vi "AWG not-simple.vi"() -> ()   [LabVIEW 2015]
uses:
  <instrlib>/niFgen/niFgen.llb/niFgen Output Mode.ctl
  <instrlib>/niFgen/niFgen.llb/niFgen Create Waveform (WDT).vi
panel:
  in  "Element":enum32{"Radio Selection 1", "Radio Selection 2"}(radio)
  in  "Save Current Waveform":bool
  in  "Load Saved Waveform":bool
  in  "Stable  Measurement":bool
  in  "Stable 2":sgl(slide) min=0 max=10 step=0.001 scale=0.0..10.0
  in  "Stable":sgl(slide) min=0 max=10 step=0.001 scale=0.0..10.0
  in  "Rare":sgl(slide) min=0 max=10 step=0.001 scale=0.0..10.0
  in  "Tab Control":T1(tab)
  in  "Calculate Rare \nFrom Stable":bool
  in  "Stop 2":bool
  in  "Apply Settings":bool
  out "Waveform Chart 3":waveform(dbl)(graph)
  in  "Tuning Isotope":enum32{"Stable 1", "Stable 2", "Rare"}(radio)
  in  "Stable 2 window (ms)":dbl=0.1
  out "Stable 2 Samples":dbl
  in  "Create New Waveform":bool
  out "Waveform Chart 2":waveform(dbl)(graph)
  in  "Bounce Field Frequency (Hz)":dbl=10.0
  in  "Waveform Samples":dbl=100000.0
  out "Waveform Period (ms)":dbl
  out "Waveform File Size (MB)":dbl
  in  "Stable window (ms)":dbl=0.1
  out "Rare Window (ms)":dbl
  out "Stable Samples":dbl
  out "Rare Samples":dbl
  out "delta-T":dbl
  in  "Stop":bool
  in  "Apply Changes":bool
  out "Sample Rate":dbl
  in  "Resource Name":refnum<k15>="ArbWaveformGen"
  out "Error Report":errorcluster
  in  "User Gain":dbl=10.0
  in  "FGEN Gain":dbl=5.0
  in  "Bytes/Sample":dbl=2.0
  # "Stable - Stable"
  # "Single Stable"
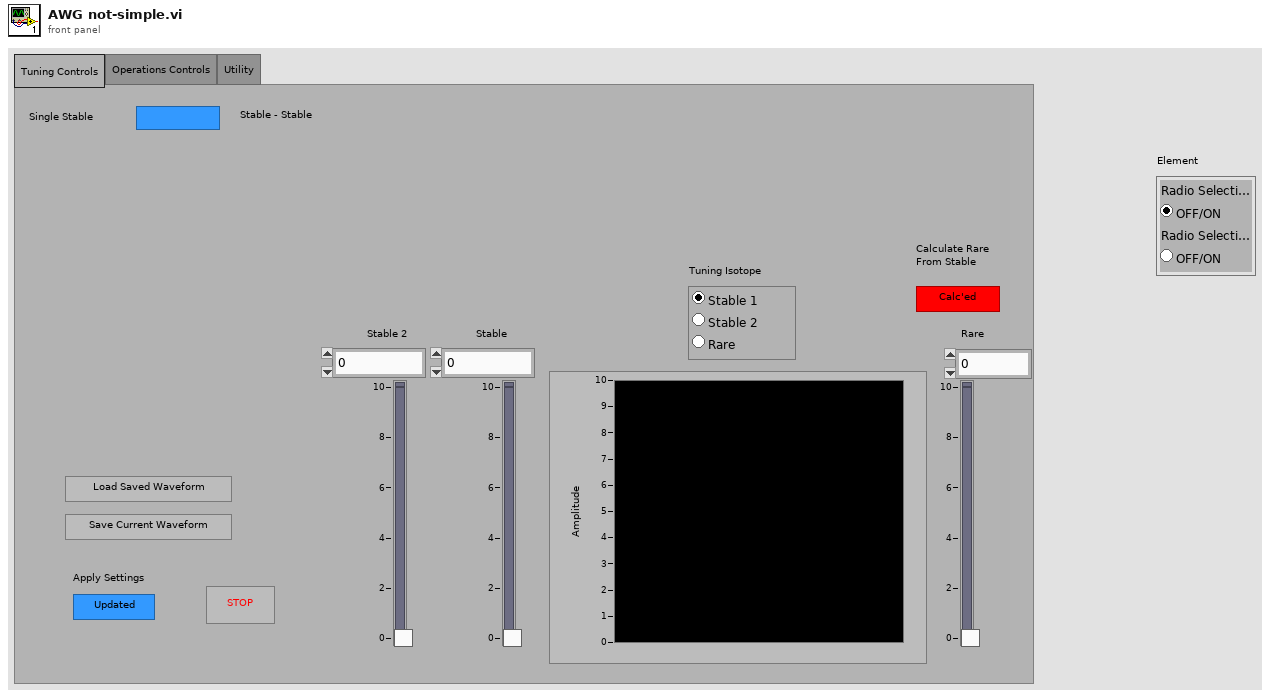
[diagram p1: front panel]
types:
  T1 = enum32{"Tuning Controls", "Operations Controls", "Utility"}
  T2 = enum8{"Enabled", "Disabled", "Disabled and Grayed Out"}
  T3 = typedef "niFgen Output Mode.ctl" = u32
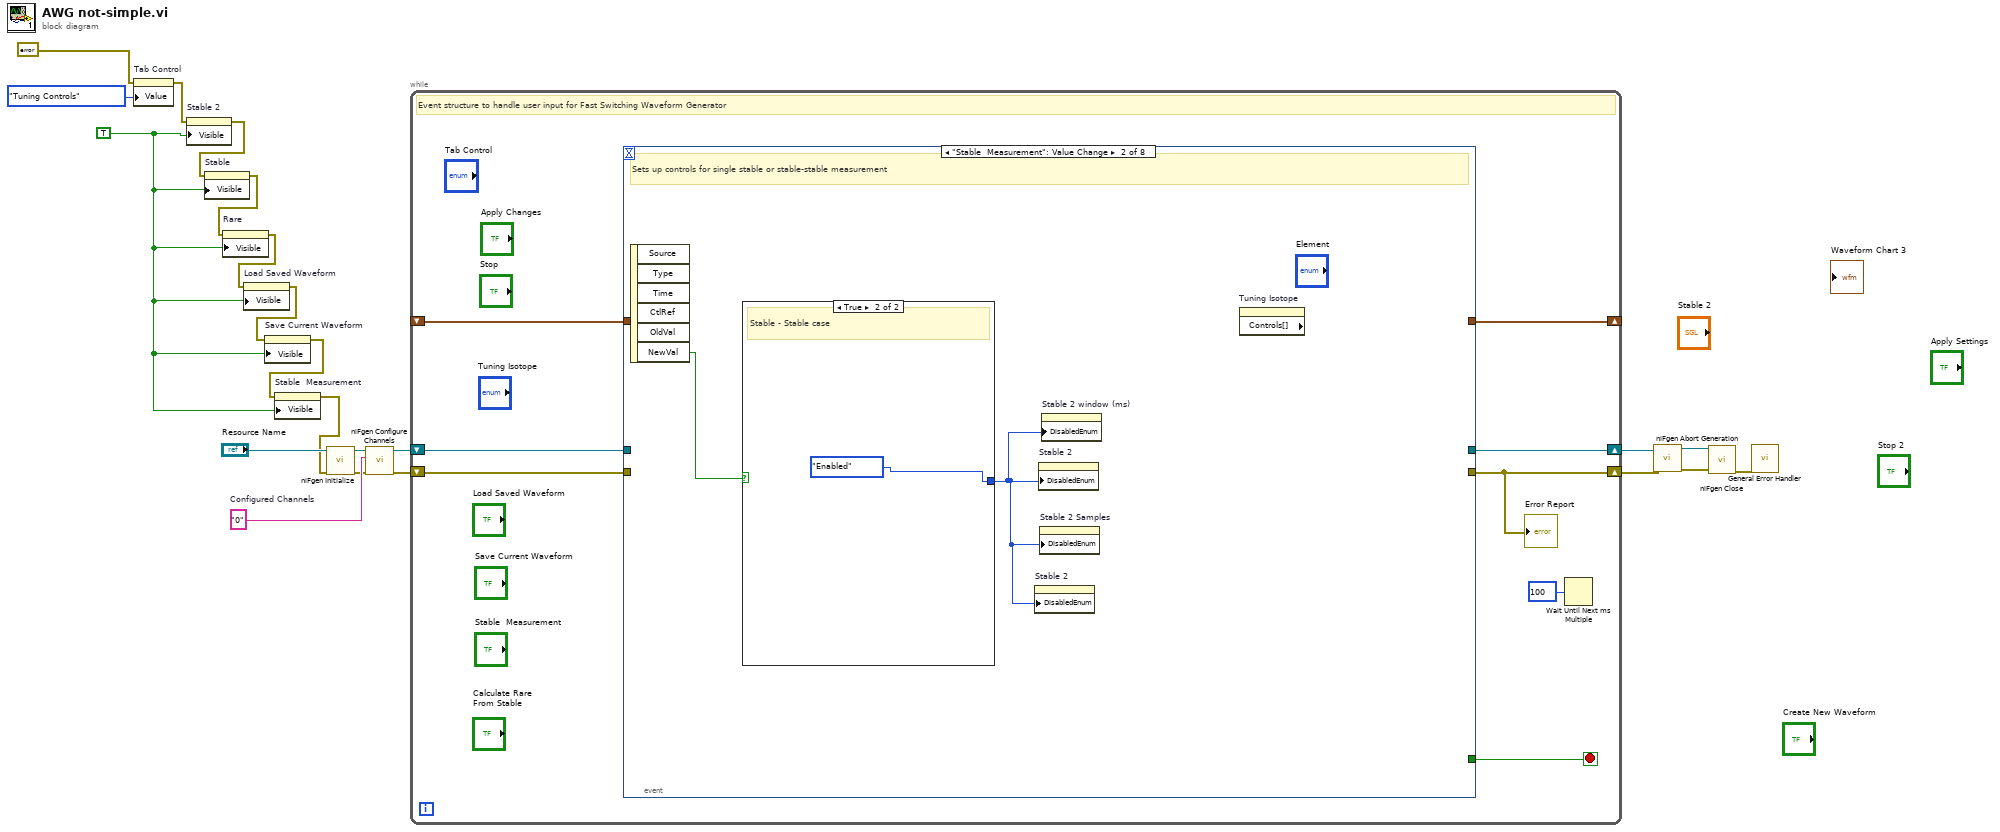
[diagram p0: block diagram]
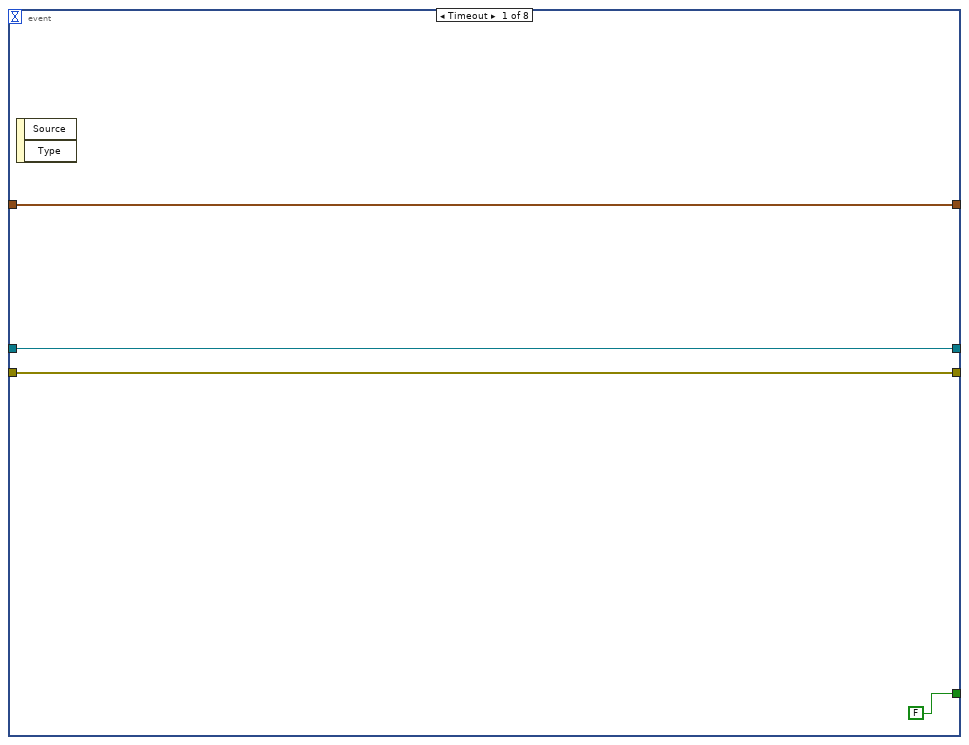
[diagram p2: hidden frame]
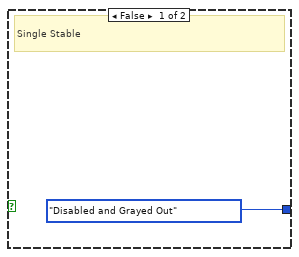
[diagram p3: hidden frame]
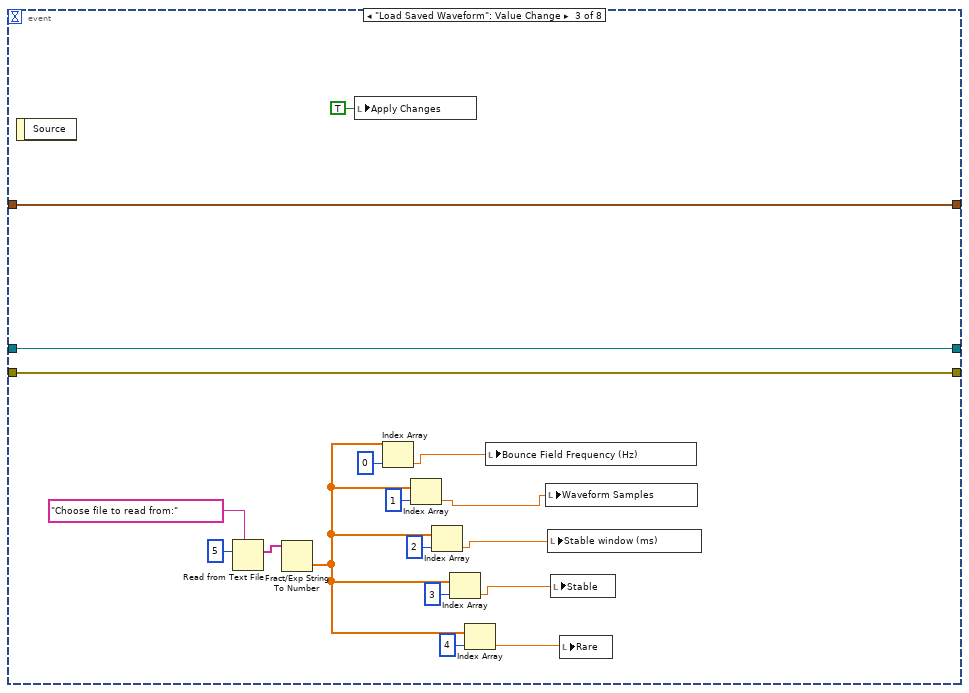
[diagram p4: hidden frame]
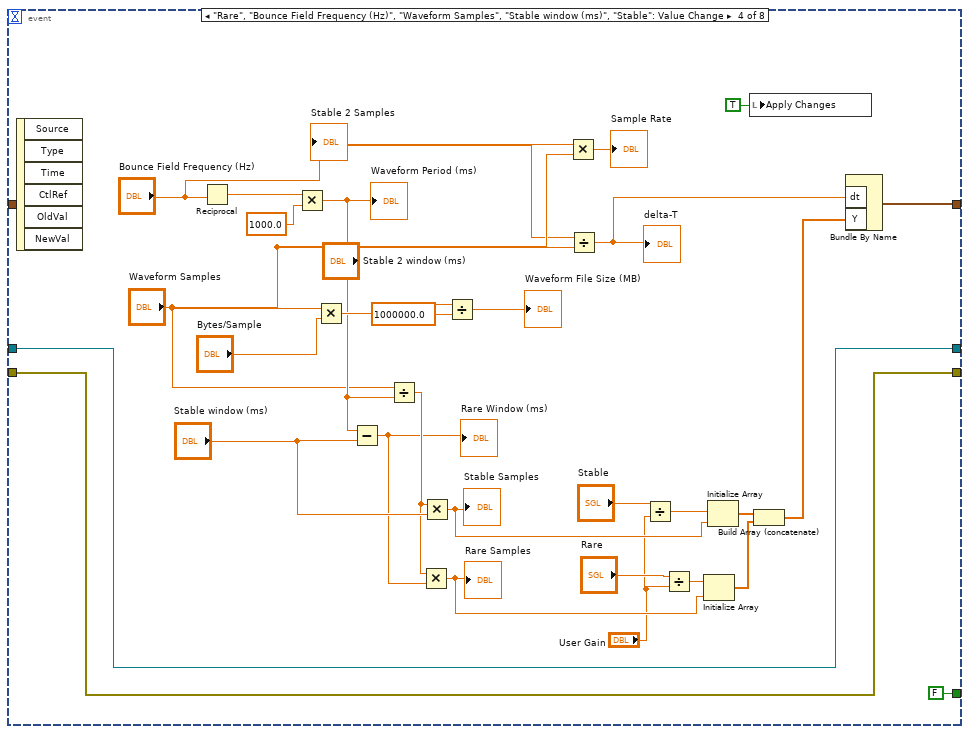
[diagram p5: hidden frame]
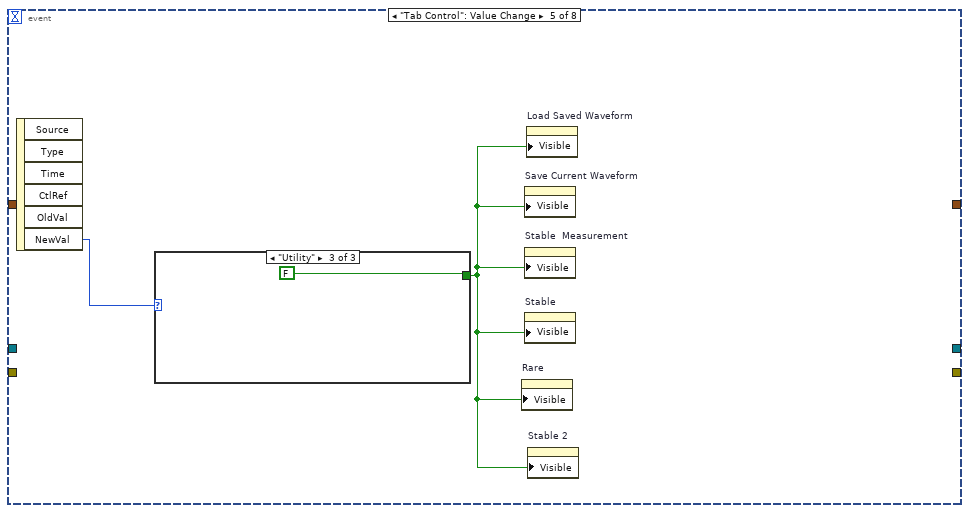
[diagram p6: hidden frame]
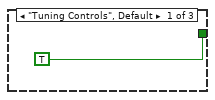
[diagram p7: hidden frame]
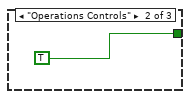
[diagram p8: hidden frame]
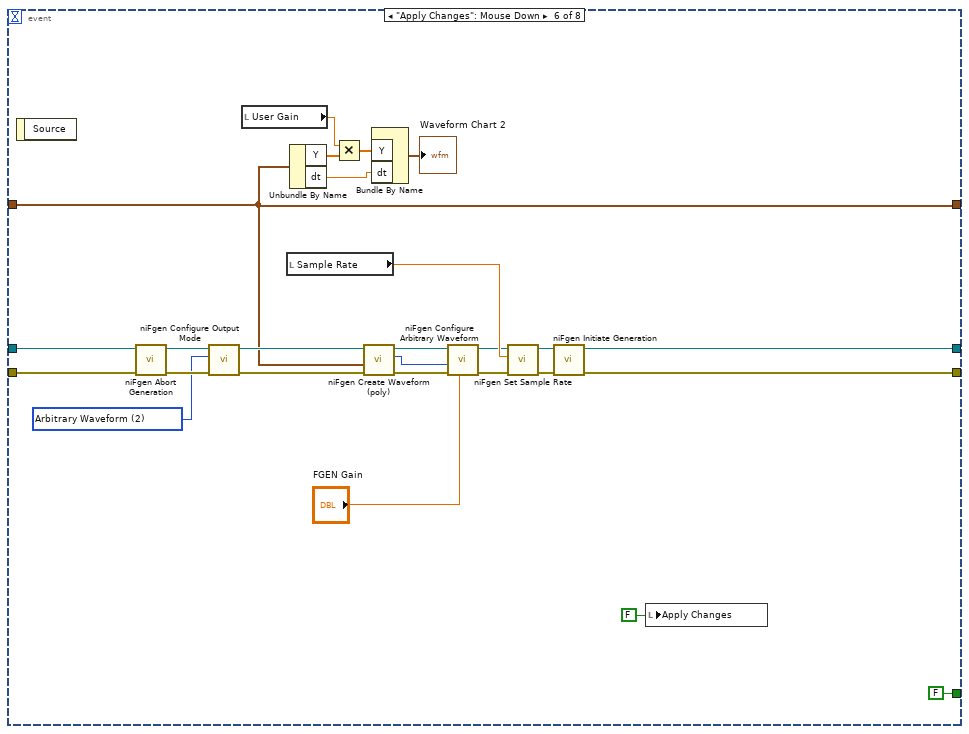
[diagram p9: hidden frame]
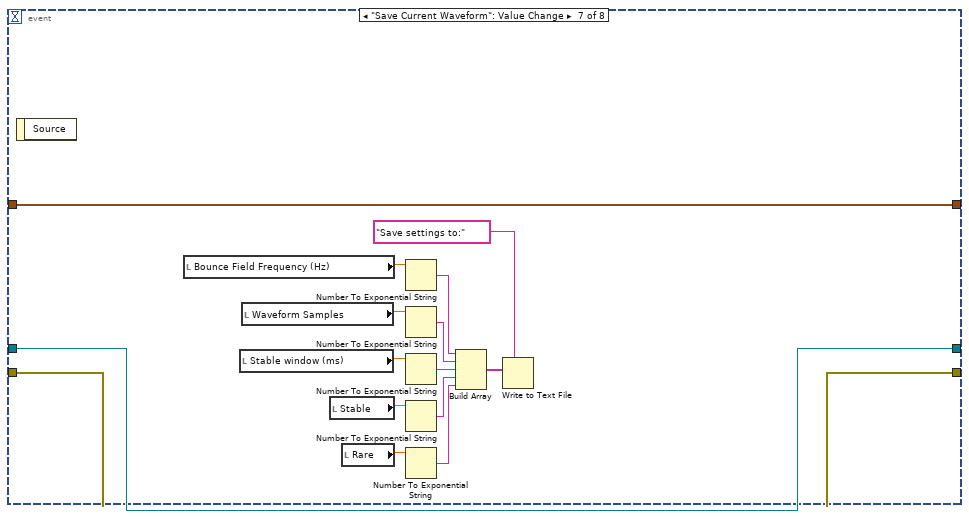
[diagram p10: hidden frame]
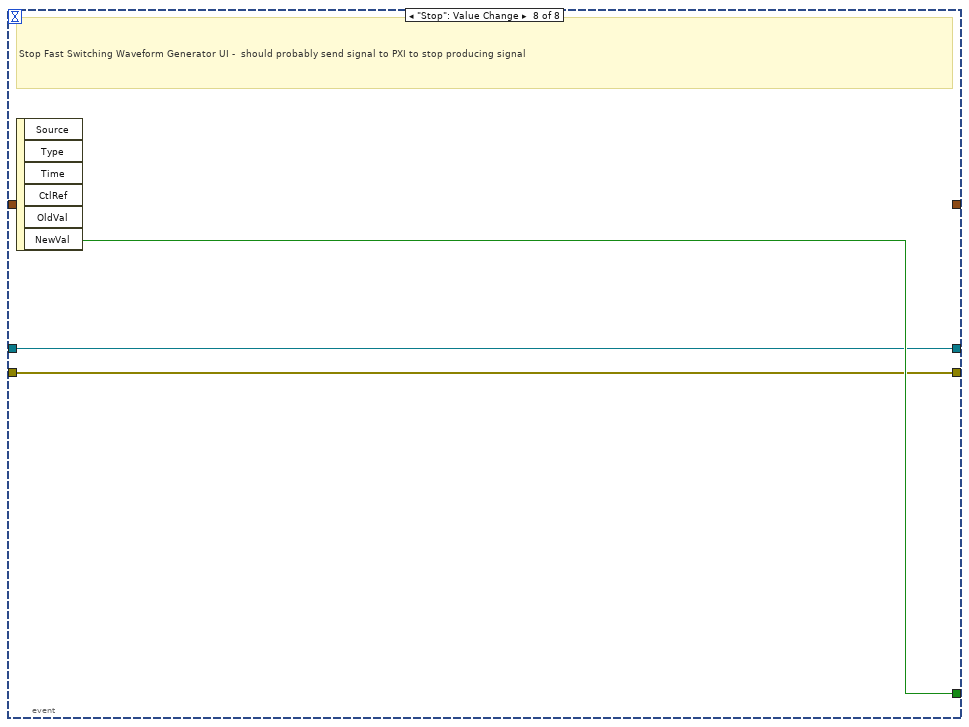
[diagram p11: hidden frame]
diagram:
  w1 = TRUE
  w20 = "0"  # Configured Channels
  n1 = property on="Tab Control" class="TabCtl (strict)"(error in=errorcluster {"status"=FALSE, "code"=0, "source"=""} ("error in (no error)"), "Value"=T1."Tuning Controls" ("Tab Control")) -> (error out=w7:errorcluster)  [unwired: 1 in, 1 out]
  n2 = property on="Stable 2" class="Slide (strict)"(error in=w7, "Visible"=w1) -> (error out=w6:errorcluster)  [unwired: 1 in, 1 out]
  n3 = property on="Stable" class="Slide (strict)"(error in=w6, "Visible"=w1) -> (error out=w5:errorcluster)  [unwired: 1 in, 1 out]
  n4 = property on="Rare" class="Slide (strict)"(error in=w5, "Visible"=w1) -> (error out=w4:errorcluster)  [unwired: 1 in, 1 out]
  n5 = property on="Load Saved Waveform" class="Bool"(error in=w4, "Visible"=w1) -> (error out=w3:errorcluster)  [unwired: 1 in, 1 out]
  n6 = property on="Save Current Waveform" class="Bool"(error in=w3, "Visible"=w1) -> (error out=w2:errorcluster)  [unwired: 1 in, 1 out]
  n7 = property on="Stable  Measurement" class="Bool (strict)"(error in=w2, "Visible"=w1) -> (error out=w10:errorcluster)  [unwired: 1 in, 1 out]
  n8 = call <instrlib>:"niFgen Initialize.vi"("error in (no error)"=w10, "Resource Name"="Resource Name") -> ("error out"=w19:errorcluster, "Instrument Handle Out"=w18:refnum<k15>)  [unwired: 8 in]
  n9 = call <instrlib>:"niFgen Configure Channels.vi"("error in (no error)"=w19, "Channels"=w20, "Instrument Handle"=w18) -> ("error out"=w15:errorcluster, "Instrument Handle Out"=w16:refnum<k15>)  [unwired: 7 in]
  n10 = while {
    shift-right: [w29] -> _
    shift-left: _ -> [w28]
    shift-right: [w22] -> w14
    shift-left: w16 -> [w24]
    shift-right: [w23] -> w13
    shift-left: w15 -> [w25]
    stop <- w26 stop-if-true
    # "Event structure to handle user input for Fast Switching Waveform Generator"
    n11 = event shown="[1] \"Stable  Measurement\": Value Change" {
      selector: _ -> [_ _ _ _ _ _ _ _]
      dyn-events: _ -> [_ _ _ _ _ _ _ _]
      timeout: _ -> [_ _ _ _ _ _ _ _]
      tunnel: [w33 _ w40 w69 _ w95 w130 _] -> w29
      tunnel: w28 -> [w33 _ w40 _ _ w95 w130 _]
      tunnel: [FALSE ("NewVal") _ _ FALSE ("stop") _ FALSE ("stop") _ w133] -> w26
      tunnel: w25 -> [w30 _ w38 w66 _ w99 w117 w132]
      tunnel: w24 -> [w31 _ w39 w65 _ w100 w116 w131]
      tunnel: [w30 _ w38 w66 _ w113 w117 w132] -> w23
      tunnel: [w31 _ w39 w65 _ w112 w116 w131] -> w22
      event Timeout {
        n12 = event-data() -> ()  [unwired: 1 in, 2 out]
      }
      event "Stable  Measurement": Value Change {
        # "Sets up controls for single stable or stable-stable measurement"
        n13 = event-data() -> ("NewVal"=w35:bool)  [unwired: 1 in, 5 out]
        n14 = case shown="True" w35 {
          tunnel: [T2."Disabled and Grayed Out" ("Disabled") T2."Enabled" ("Disabled")] -> w34
          frame False {
            # "Single Stable"
          }
          frame True {
            # "Stable - Stable case"
          }
        }
        n15 = property on="Stable 2" class="Bool (strict)"("DisabledEnum"=w34) -> ()  [unwired: 2 in, 2 out]
        n16 = property on="Stable 2" class="Slide (strict)"("DisabledEnum"=w34) -> ()  [unwired: 2 in, 2 out]
        n17 = property on="Stable 2 Samples" class="DigNum (strict)"("DisabledEnum"=w34) -> ()  [unwired: 2 in, 2 out]
        n18 = property on="Stable 2 window (ms)" class="DigNum (strict)"("DisabledEnum"=w34) -> ()  [unwired: 2 in, 2 out]
        n19 = property on="Tuning Isotope" class="RadioBtnsControl (strict)" props=["Controls[]"]() -> ()  [unwired: 2 in, 3 out]
      }
      event "Load Saved Waveform": Value Change {
        n20 = event-data() -> ()  [unwired: 1 in, 1 out]
        n21 = Read from Text File(prompt (Open existing file)="Choose file to read from:", count=5) -> (text=w53:string[])  [unwired: 2 in, 3 out]
        n22 = Fract/Exp String To Number(string=w53) -> (number=w46:dbl[])  [unwired: 3 in, 1 out]
        n23 = local write "Apply Changes"(TRUE ("Apply Changes")) -> ()
        n24 = Index Array(array=w46, index=0) -> (element=w51:dbl)
        n25 = Index Array(array=w46, index=1) -> (element=w47:dbl)
        n26 = Index Array(array=w46, index=2) -> (element=w48:dbl)
        n27 = Index Array(array=w46, index=3) -> (element=w49:dbl)
        n28 = Index Array(array=w46, index=4) -> (element=w50:dbl)
        n29 = local write "Bounce Field Frequency (Hz)"(w51) -> ()
        n30 = local write "Waveform Samples"(w47) -> ()
        n31 = local write "Stable window (ms)"(w48) -> ()
        n32 = local write "Stable"(w49) -> ()
        n33 = local write "Rare"(w50) -> ()
      }
      event "Rare", "Bounce Field Frequency (Hz)", "Waveform Samples", "Stable window (ms)", "Stable": Value Change {
        n34 = event-data() -> ()  [unwired: 1 in, 6 out]
        n35 = Reciprocal(x="Bounce Field Frequency (Hz)") -> (1/x=w64:dbl)
        n36 = Multiply(x=w64, y=1000.0) -> (x*y=w72:dbl)
        "Waveform Period (ms)" <- w72
        n37 = Multiply(x="Waveform Samples", y="Bytes/Sample") -> (x*y=w79:dbl)
        n38 = Subtract(x=w72, y="Stable window (ms)") -> (x-y=w81:dbl)
        "Rare Window (ms)" <- w81
        n39 = Divide(x="Waveform Samples", y=w72) -> (x/y=w82:dbl)
        n40 = Multiply(x=w82, y=w81) -> (x*y=w75:dbl)
        "Rare Samples" <- w75
        n41 = Multiply(x=w82, y="Stable window (ms)") -> (x*y=w76:dbl)
        "Stable Samples" <- w76
        n42 = Divide(x=w79, y=1000000.0) -> (x/y=→"Waveform File Size (MB)":dbl)
        n43 = Multiply(x="Bounce Field Frequency (Hz)", y="Waveform Samples") -> (x*y=→"Sample Rate":dbl)
        n44 = Divide(x="Bounce Field Frequency (Hz)", y="Waveform Samples") -> (x/y=w70:dbl)
        "delta-T" <- w70
        n45 = Divide(x="Stable", y="User Gain") -> (x/y=w61:dbl)
        n46 = Divide(x="Rare", y="User Gain") -> (x/y=w59:dbl)
        n47 = Initialize Array(w59, w75) -> (w73:dbl[])
        n48 = Initialize Array(w61, w76) -> (w74:dbl[])
        n49 = local write "Apply Changes"(TRUE ("Apply Changes")) -> ()
        n50 = Build Array (concatenate)(w74, w73) -> (w71:dbl[])
        n51 = Bundle By Name("dt"=w70, "Y"=w71) -> (w69:waveform(dbl))  [unwired: 1 in]
      }
      event "Tab Control": Value Change {
        n52 = event-data() -> ("NewVal"=w86:T1)  [unwired: 1 in, 5 out]
        n53 = case shown="\"Utility\"" w86 {
          tunnel: [TRUE ("Visible") TRUE ("Visible") FALSE ("Visible")] -> w85
          frame "Tuning Controls", Default {
          }
          frame "Operations Controls" {
          }
          frame "Utility" {
          }
        }
        n54 = property on="Rare" class="Slide (strict)"("Visible"=w85) -> ()  [unwired: 2 in, 2 out]
        n55 = property on="Save Current Waveform" class="Bool"("Visible"=w85) -> ()  [unwired: 2 in, 2 out]
        n56 = property on="Stable  Measurement" class="Bool (strict)"("Visible"=w85) -> ()  [unwired: 2 in, 2 out]
        n57 = property on="Stable" class="Slide (strict)"("Visible"=w85) -> ()  [unwired: 2 in, 2 out]
        n58 = property on="Load Saved Waveform" class="Bool"("Visible"=w85) -> ()  [unwired: 2 in, 2 out]
        n59 = property on="Stable 2" class="Slide (strict)"("Visible"=w85) -> ()  [unwired: 2 in, 2 out]
      }
      event "Apply Changes": Mouse Down {
        w101 = T3 2 items=["Standard Function", "Frequency List", "Arbitrary Waveform", "Arbitrary Sequence", "Script"] ("Output Mode (default: 0=Standard Function)")
        n60 = event-data() -> ()  [unwired: 1 in, 1 out]
        n61 = call <instrlib>:"niFgen Abort Generation.vi"("error in (no error)"=w99, "Instrument Handle"=w100) -> ("error out"=w102:errorcluster, "Instrument Handle Out"=w103:refnum<k15>)  [unwired: 8 in]
        n62 = call <instrlib>:"niFgen Configure Output Mode.vi"("error in (no error)"=w102, "Output Mode (default: 0=Standard Function)"=w101, "Instrument Handle"=w103) -> ("error out"=w97:errorcluster, "Instrument Handle Out"=w98:refnum<k15>)  [unwired: 6 in]
        n63 = local read "User Gain"() -> (w91:dbl)
        n64 = local read "Sample Rate"() -> (w108:dbl)
        n65 = Unbundle By Name(w95) -> ("Y"=w92:dbl[], "dt"=w94:dbl)
        n66 = Multiply(x=w91, y=w92) -> (x*y=w93:dbl[])
        n67 = call-poly <instrlib>:"niFgen Create Waveform (poly).vi"("error in (no error)"=w97, "Waveform"=w95, "Instrument Handle"=w98) -> ("error out"=w104:errorcluster, "Waveform Handle"=w106:i32, "Instrument Handle Out"=w111:refnum<k15>)  [unwired: 6 in]
        n68 = Bundle By Name("Y"=w93, "dt"=w94) -> (→"Waveform Chart 2":waveform(dbl))  [unwired: 1 in]
        n69 = call <instrlib>:"niFgen Configure Arbitrary Waveform.vi"("Gain"="FGEN Gain", "error in (no error)"=w104, "Waveform Handle"=w106, "Instrument Handle"=w111) -> ("error out"=w105:errorcluster, "Instrument Handle Out"=w107:refnum<k15>)  [unwired: 6 in]
        n70 = call <instrlib>:"niFgen Set Sample Rate.vi"("error in (no error)"=w105, "Sample Rate (Samp/s)"=w108, "Instrument Handle"=w107) -> ("error out"=w109:errorcluster, "Instrument Handle Out"=w110:refnum<k15>)  [unwired: 7 in]
        n71 = call <instrlib>:"niFgen Initiate Generation.vi"("error in (no error)"=w109, "Instrument Handle"=w110) -> ("error out"=w113:errorcluster, "Instrument Handle Out"=w112:refnum<k15>)  [unwired: 8 in]
        n72 = local write "Apply Changes"(FALSE ("Apply Changes")) -> ()
      }
      event "Save Current Waveform": Value Change {
        n73 = event-data() -> ()  [unwired: 1 in, 1 out]
        n74 = local read "Bounce Field Frequency (Hz)"() -> (w129:dbl)
        n75 = local read "Stable window (ms)"() -> (w125:dbl)
        n76 = local read "Waveform Samples"() -> (w126:dbl)
        n77 = local read "Stable"() -> (w128:sgl)
        n78 = local read "Rare"() -> (w127:sgl)
        n79 = Number To Exponential String(number=w129) -> (E-format string=w124:string)  [unwired: 3 in]
        n80 = Number To Exponential String(number=w126) -> (E-format string=w121:string)  [unwired: 3 in]
        n81 = Number To Exponential String(number=w125) -> (E-format string=w120:string)  [unwired: 3 in]
        n82 = Number To Exponential String(number=w128) -> (E-format string=w119:string)  [unwired: 3 in]
        n83 = Number To Exponential String(number=w127) -> (E-format string=w118:string)  [unwired: 3 in]
        n84 = Build Array(w124, w121, w120, w119, w118) -> (w123:string[])
        n85 = Write to Text File(prompt (Choose or enter file path)="Save settings to:", text=w123) -> ()  [unwired: 2 in, 3 out]
      }
      event "Stop": Value Change {
        # "Stop Fast Switching Waveform Generator UI -  should probably send signal to PXI to stop producing signal"
        n86 = event-data() -> ("NewVal"=w133:bool)  [unwired: 1 in, 5 out]
      }
    }
    "Error Report" <- w23
    n87 = Wait Until Next ms Multiple(millisecond multiple=u32 100) -> ()  [unwired: 1 out]
  }
  n88 = call <instrlib>:"niFgen Abort Generation.vi"("error in (no error)"=w13, "Instrument Handle"=w14) -> ("error out"=w12:errorcluster, "Instrument Handle Out"=w11:refnum<k15>)  [unwired: 8 in]
  n89 = call <instrlib>:"niFgen Close.vi"("error in (no error)"=w12, "Instrument Handle"=w11) -> ("error out"=w17:errorcluster)  [unwired: 9 in]
  n90 = call <vilib>:"General Error Handler.vi"("error in (no error)"=w17) -> ()  [unwired: 10 in, 5 out]
